vi "Image To EDVR同元素地址操作.vi"() -> ()   [LabVIEW 2014]
doc: "This example shows how to convert an image into a two-dimensional LabVIEW External Data Value Reference (EDVR). By converting an image into an EDVR and using the In Place Element Structure, you can apply all the analysis, display, and array operators available in LabVIEW to the image data. These operations can be done directly on the image pixel data without have to copy the image data into a temporary array.\n\nIn this example two images (Image To EDVR Image and Merge Image) are merged together using Logarithmic Image Processing (LIP) addition and written written back to the Image To EDVR Image. Follow the template provided in this example to properly synchronize EDVR accesses with other Vision Development Module operations and image displays. Use the error handling model provided to ensure that any errors will be collected properly."
uses:
  <vilib>/vision/EDVR.llb/IMAQ ImageToEDVR 2D U8.vi
panel:
  out "Image Result":T1(plugin-control)
  out "Merge Image":T1(plugin-control)
  out "Image Source":T1(plugin-control)
  # "Overview: Demonstrates how to retrieve and use an External Data Value Reference (EDVR) of the pixel values from an image by merging the two images on the left to form the Image Result on the right.\nRequirements: NI Vision Development Module\nInstructions: Run the VI."
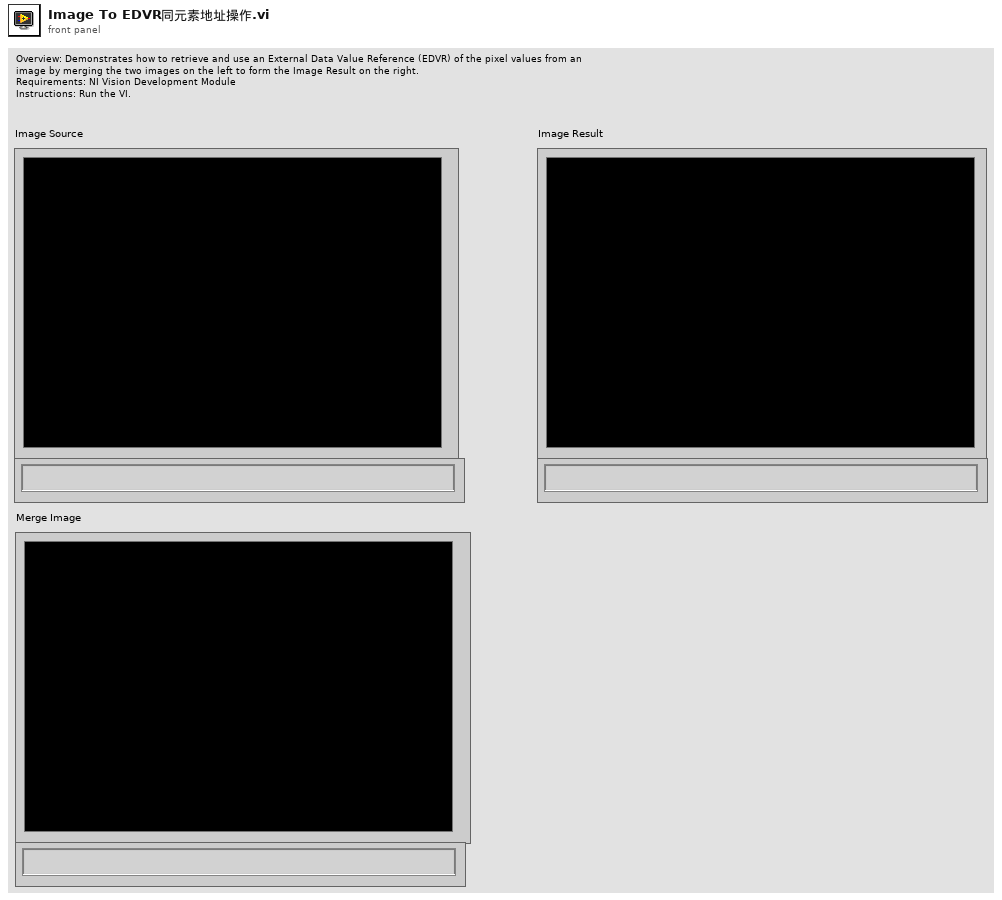
[diagram p1: front panel]
types:
  T1 = typedef "IMAQ Image.ctl" = refnum<image>
  T2 = typedef "Image Type" = u32
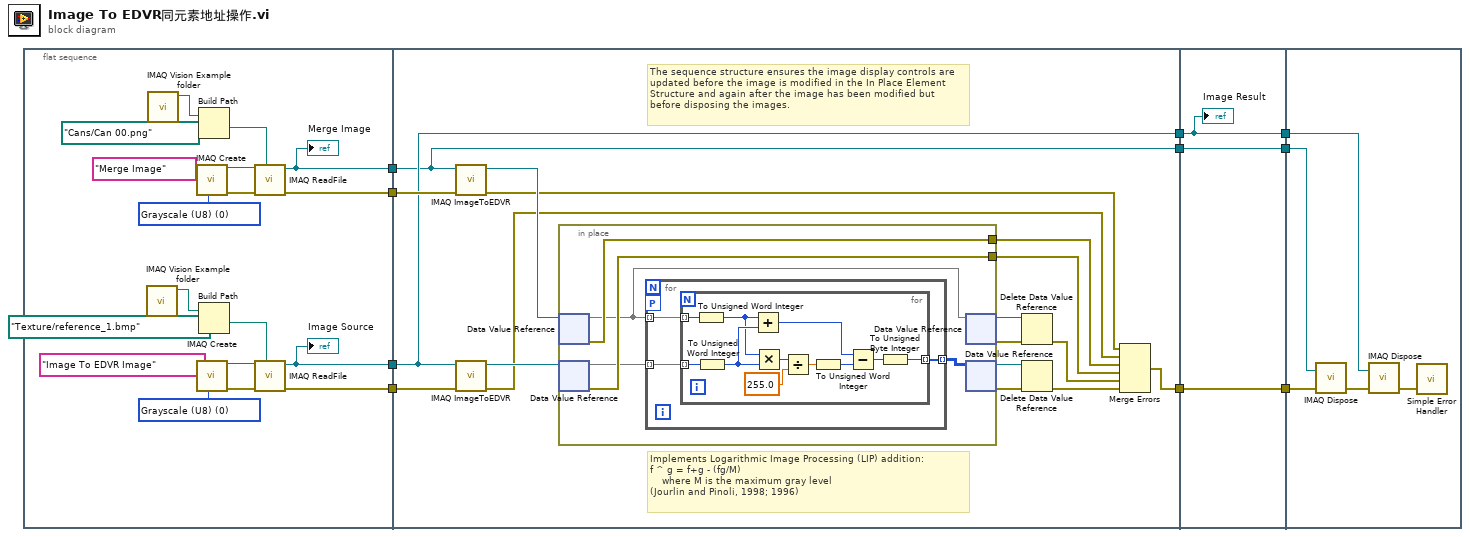
[diagram p0: block diagram]
diagram:
  n1 = flat-sequence {
    tunnel: [w16] -> w8
    tunnel: [w15] -> w7
    tunnel: [w14] -> w6
    tunnel: [w13] -> w5
    tunnel: [w41] -> w10
    tunnel: w8 -> [w30]
    tunnel: w7 -> [w32]
    tunnel: w6 -> [w31]
    tunnel: w5 -> [w29]
    tunnel: [w30] -> w4
    tunnel: [w29] -> w3
    tunnel: w10 -> [w67]
    tunnel: [w67] -> w9
    tunnel: w4 -> [w65]
    tunnel: w3 -> [w66]
    tunnel: [w66] -> w2
    tunnel: [w65] -> w1
    tunnel: w9 -> [w71]
    tunnel: w2 -> [w69]
    tunnel: w1 -> [w68]
    frame #0 {
      w23 = T2 0 items=["Grayscale (U8)", "Grayscale (I16)", "Grayscale (SGL)", "Complex (CSG)", "RGB (U32)", "HSL (U32)", "RGB (U64)", "Grayscale (U16)"] ("Image Type")
      w22 = T2 0 items=["Grayscale (U8)", "Grayscale (I16)", "Grayscale (SGL)", "Complex (CSG)", "RGB (U32)", "HSL (U32)", "RGB (U64)", "Grayscale (U16)"] ("Image Type")
      n2 = call "IMAQ Vision Example folder.vi"() -> ("Example Image Path"=w18:path)  [unwired: 11 in]
      n3 = call "IMAQ Vision Example folder.vi"() -> ("Example Image Path"=w27:path)  [unwired: 11 in]
      n4 = call "IMAQ Create"("Image Name"="Merge Image", "Image Type"=w23) -> ("New Image"=w25:T1, "error out"=w26:errorcluster)  [unwired: 3 in]
      n5 = call "IMAQ Create"("Image Name"="Image To EDVR Image", "Image Type"=w22) -> ("New Image"=w20:T1, "error out"=w19:errorcluster)  [unwired: 3 in]
      n6 = Build Path(base path=w27, name or relative path=path "Cans/Can 00.png") -> (appended path=w24:path)
      n7 = Build Path(base path=w18, name or relative path=path "Texture/reference_1.bmp") -> (appended path=w21:path)
      n8 = call "IMAQ ReadFile"("File Path"=w24, "error in (no error)"=w26, "Image"=w25) -> ("error out"=w14:errorcluster, "Image Out"=w13:T1)  [unwired: 4 in, 3 out]
      "Merge Image" <- w13
      n9 = call "IMAQ ReadFile"("File Path"=w21, "error in (no error)"=w19, "Image"=w20) -> ("error out"=w15:errorcluster, "Image Out"=w16:T1)  [unwired: 4 in, 3 out]
      "Image Source" <- w16
    }
    frame #1 {
      # "Implements Logarithmic Image Processing (LIP) addition:\nf ^ g = f+g - (fg/M)\n    where M is the maximum gray level\n(Jourlin and Pinoli, 1998; 1996)"
      # "The sequence structure ensures the image display controls are updated before the image is modified in the In Place Element Structure and again after the image has been modified but  before disposing the images."
      n10 = call-poly <vilib>:"IMAQ ImageToEDVR.vi"("error in (no error)"=w31, "Image"=w29) -> ("error out"=w36:errorcluster, "EDVR 2D U8"=w40:refnum<data-value>)  [unwired: 7 in, 1 out]
      n11 = call-poly <vilib>:"IMAQ ImageToEDVR.vi"("error in (no error)"=w32, "Image"=w30) -> ("error out"=w37:errorcluster, "EDVR 2D U8"=w42:refnum<data-value>)  [unwired: 7 in, 1 out]
      n12 = in-place {
        in-place-border: [w50] -> w39
        in-place-border: [w47] -> w38
        n13 = in-place-dvr #1(w40) -> (w46:u8[][], w47:errorcluster)
        n14 = in-place-dvr #2(w42) -> (w49:u8[][], w50:errorcluster)
        n15 = for {
          tunnel: w46 -> [w53] mode=indexing
          tunnel: w49 -> [w52] mode=indexing
          tunnel: [w51] -> w48 mode=indexing
          workers-P: _ -> [_]
          n16 = for {
            tunnel: w53 -> [w62] mode=indexing
            tunnel: w52 -> [w63] mode=indexing
            tunnel: [w60] -> w51 mode=indexing
            n17 = To Unsigned Word Integer(number=w62) -> (unsigned 16bit integer=w54:u16)
            n18 = To Unsigned Word Integer(number=w63) -> (unsigned 16bit integer=w55:u16)
            n19 = Add(x=w54, y=w55) -> (x+y=w64:u16)
            n20 = Multiply(x=w54, y=w55) -> (x*y=w59:u16)
            n21 = Divide(x=w59, y=255.0) -> (x/y=w57:dbl)
            n22 = To Unsigned Word Integer(number=w57) -> (unsigned 16bit integer=w56:u16)
            n23 = Subtract(x=w64, y=w56) -> (x-y=w61:u16)
            n24 = To Unsigned Byte Integer(number=w61) -> (unsigned 8bit integer=w60:u8)
          }
        }
        n25 = in-place-dvr #1(w46) -> (w34:refnum<data-value>, w35:errorcluster)
        n26 = in-place-dvr #2(w48) -> (w44:refnum<data-value>, w43:errorcluster)
      }
      n27 = Delete Data Value Reference(data value reference=w34, error in=w35) -> (error out=w33:errorcluster)  [unwired: 1 out]
      n28 = Delete Data Value Reference(data value reference=w44, error in=w43) -> (error out=w45:errorcluster)  [unwired: 1 out]
      n29 = Merge Errors(w36, w37, w38, w39, w33, w45) -> (w41:errorcluster)
    }
    frame #2 {
      "Image Result" <- w65
    }
    frame #3 {
      n30 = call "IMAQ Dispose"("Image"=w69, "error in (no error)"=w71) -> ("error out"=w70:errorcluster)  [unwired: 4 in]
      n31 = call "IMAQ Dispose"("Image"=w68, "error in (no error)"=w70) -> ("error out"=w72:errorcluster)  [unwired: 4 in]
      n32 = call <vilib>:"Simple Error Handler.vi"("error in (no error)"=w72) -> ()  [unwired: 4 in, 5 out]
    }
  }
